vi "Write Position.vi"(8 "error in (no error)":errorcluster, 10 "Position":T1, 11 "Fortress in":refnum<class "Fortress.lvclass">) -> (0 "error out":errorcluster, 3 "Fortress out":refnum<class "Fortress.lvclass">)   [LabVIEW 2015, in "Fortress.lvclass"]
uses:
  Fortress.lvclass
  Common/Position.ctl
  Fortress.lvclass/Fortress.ctl
  Common/Common.lvlib
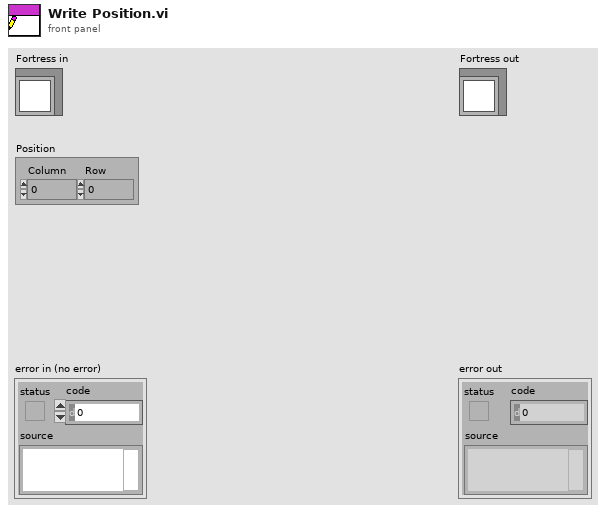
[diagram p1: front panel]
types:
  T1 = typedef "Common.lvlib/Position.ctl" = cluster{"Column":i32, "Row":i32}
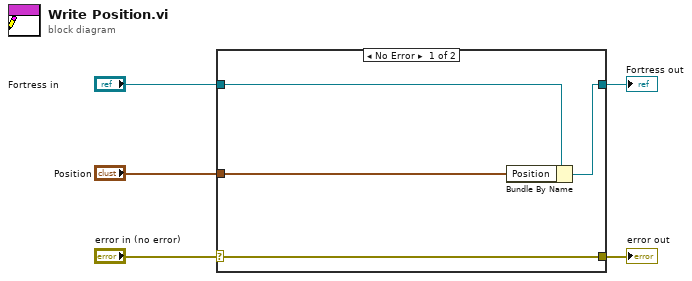
[diagram p0: block diagram]
diagram:
  n1 = case shown="No Error" "error in (no error)" {
    selector: "error in (no error)" -> [w9 w10]
    tunnel: [w9 w10] -> w4
    tunnel: [w7 w11] -> w2
    tunnel: "Fortress in" -> [w8 w11]
    tunnel: "Position" -> [w6 _]
    frame No Error {
      n2 = Bundle By Name(cluster=w8, "Position"=w6) -> (w7:refnum<class "Fortress.lvclass">)
    }
    frame Error {
    }
  }
  "error out" <- w4
  "Fortress out" <- w2
